vi "Another single shot try.vi"(8 "Error In":errorcluster, 11 "Camera reference in":refnum<k24>) -> (0 "Error Out":errorcluster, 2 "Array":u16[][](array[numeric]), 3 "Camera reference out":refnum<k24>)   [LabVIEW 2017]
uses:
  C:/Program Files/National Instruments/LabVIEW 2017/instr.lib/IDS/ueye.NET/uEyeDotNet.dll
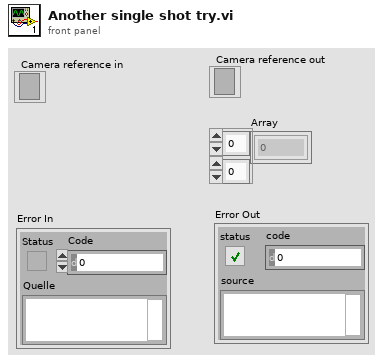
[diagram p1: front panel]
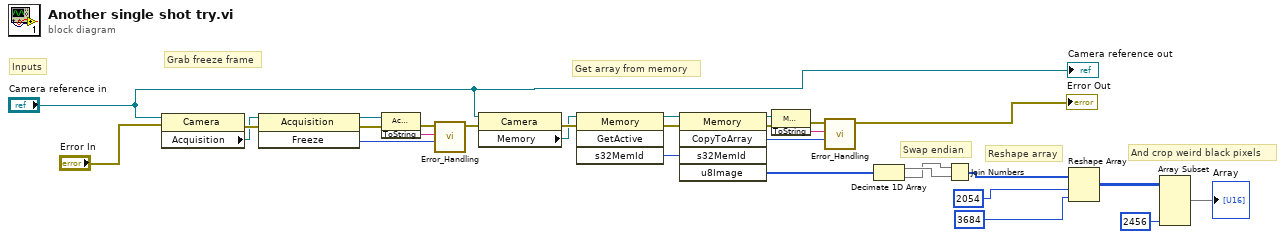
[diagram p0: block diagram]
diagram:
  # "Swap endian"
  # "And crop weird black pixels"
  # "Reshape array"
  # "Get array from memory"
  # "Grab freeze frame"
  # "Inputs"
  n1 = property class="Camera"(reference="Camera reference in", error in="Error In") -> (error out=w24:errorcluster, "Acquisition"=w23:refnum<k24>)  [unwired: 1 out]
  n2 = invoke class="Acquisition" method="Freeze"(reference=w23, error in=w24) -> (reference out=w28:refnum<k24>, error out=w27:errorcluster, "Freeze"=w29:i32)  [unwired: 1 in]
  n3 = invoke class="Acquisition" method="ToString"(reference=w28, error in=w27) -> (error out=w25:errorcluster, "ToString"=w26:string)  [unwired: 1 in, 1 out]
  n4 = call <instrlib>:"Error_Handling.vi"("Error Code"=w29, "Error String"=w26, "Error In"=w25) -> ("Error Out"=w4:errorcluster)  [unwired: 8 in]
  n5 = property class="Camera"(reference="Camera reference in", error in=w4) -> (error out=w12:errorcluster, "Memory"=w2:refnum<k24>)  [unwired: 1 out]
  n6 = invoke class="Memory" method="GetActive"(reference=w2) -> (reference out=w1:refnum<k24>, "s32MemId"=w3:i32)  [unwired: 3 in, 2 out]
  n7 = invoke class="Memory" method="CopyToArray"(reference=w1, error in=w12, "s32MemId"=w3) -> (reference out=w9:refnum<k24>, error out=w8:errorcluster, "CopyToArray"=w7:i32, "u8Image"=w13:u8[])  [unwired: 2 in, 1 out]
  n8 = invoke class="Memory" method="ToString"(reference=w9, error in=w8) -> (error out=w11:errorcluster, "ToString"=w10:string)  [unwired: 1 in, 1 out]
  n9 = call <instrlib>:"Error_Handling.vi"("Error Code"=w7, "Error String"=w10, "Error In"=w11) -> ("Error Out"=→"Error Out":errorcluster)  [unwired: 8 in]
  n10 = Decimate 1D Array(w13) -> (w20:u8[], w15:u8[])
  n11 = Join Numbers(hi=w15, lo=w20) -> ((hi.lo)=w21:u16[])
  n12 = Reshape Array(w21, 2054 ("dimension size"), 3684 ("Width")) -> (w18:u16[][])
  n13 = Array Subset(array=w18, length (col)=2456 ("length")) -> (→"Array":u16[][])  [unwired: 3 in]
  "Camera reference out" <- "Camera reference in"
